vi "Pre Launch Init.vi"(11 "Main Window in":refnum<class "Main Window.lvclass">) -> (0 "error out":errorcluster, 3 "Main Window out":refnum<class "Main Window.lvclass">)   [LabVIEW 2021, in "Recipe.lvlib" / "Main Window.lvclass"]
doc: "Initializes the panel actor. Creates the Panel Helper.\n\n----\nPlease see the following web address for additional documentation and tutorial information:\nhttp://www.mooregoodideas.com/mgi-panel-manager/\n\nAuthor: Derek Trepanier\n\nCopyright (c) 2018, Moore Good Ideas, Inc.\n\nAll rights reserved.\n\nRedistribution and use in source and binary forms, with or without modification, are permitted provided that the following conditions are met:\n\n * Redistributions of source code must retain the above copyright notice, this list of conditions and the following disclaimer.\n * Redistributions in binary form must reproduce the above copyright notice, this list of conditions and the following disclaimer in the documentation and/or other materials provided with the distribution.\n * Neither the name of Moore Good Ideas, Inc. nor the names of its contributors may be used to endorse or promote products derived from this software without specific prior written permission.\n\nTHIS SOFTWARE IS PROVIDED BY THE COPYRIGHT HOLDERS AND CONTRIBUTORS \"AS IS\" AND ANY EXPRESS OR IMPLIED WARRANTIES, INCLUDING, BUT NOT LIMITED TO, THE IMPLIED WARRANTIES OF MERCHANTABILITY AND FITNESS FOR A PARTICULAR PURPOSE ARE DISCLAIMED. IN NO EVENT SHALL THE COPYRIGHT OWNER OR CONTRIBUTORS BE LIABLE FOR ANY DIRECT, INDIRECT, INCIDENTAL, SPECIAL, EXEMPLARY, OR CONSEQUENTIAL DAMAGES (INCLUDING, BUT NOT LIMITED TO, PROCUREMENT OF SUBSTITUTE GOODS OR SERVICES; LOSS OF USE, DATA, OR PROFITS; OR BUSINESS INTERRUPTION) HOWEVER CAUSED AND ON ANY THEORY OF LIABILITY, WHETHER IN CONTRACT, STRICT LIABILITY, OR TORT (INCLUDING NEGLIGENCE OR OTHERWISE) ARISING IN ANY WAY OUT OF THE USE OF THIS SOFTWARE, EVEN IF ADVISED OF THE POSSIBILITY OF SUCH DAMAGE."
uses:
  Main Window.lvclass
  Typedefs/Path--enum.ctl
  <vilib>/MGI/Panel Manager/Panel Actor/Panel Actor/Panel Actor.lvclass
  <vilib>/Thomas ALLIBE/Path Utilities/Path Utilities.lvlib
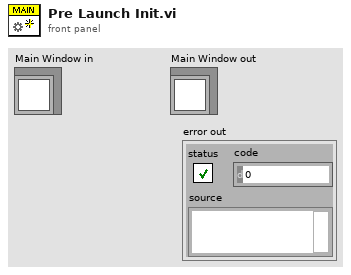
[diagram p1: front panel]
types:
  T1 = typedef "Recipe.lvlib/Main Window.lvclass/Path--enum.ctl" = enum16{"Recipe List File"}
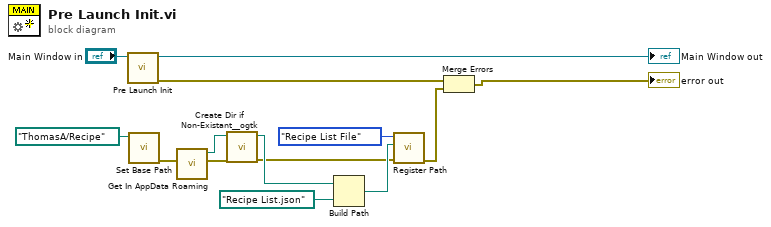
[diagram p0: block diagram]
diagram:
  n1 = call-parent "Pre Launch Init.vi"("Panel Actor in"="Main Window in") -> ("error out"=w14:errorcluster, "Panel Actor out"=→"Main Window out":refnum<class "Main Window.lvclass">)  [unwired: 9 in]
  n2 = call <vilib>:"Set Base Path.vi"("Base Path"=path "ThomasA/Recipe") -> ("error out"=w9:errorcluster)  [unwired: 9 in, 1 out]
  n3 = call <vilib>:"Get In AppData Roaming.vi"("error in (no error)"=w9) -> ("error out"=w5:errorcluster, "Path"=w4:path)  [unwired: 9 in]
  n4 = call <userlib>:"Create Dir if Non-Existant__ogtk.vi"("error in (no error)"=w5, "Directory Path"=w4) -> ("error out"=w2:errorcluster, "dup Directory Path"=w3:path)  [unwired: 7 in, 1 out]
  n5 = Build Path(base path=w3, name or relative path=path "Recipe List.json") -> (appended path=w8:path)
  n6 = call <vilib>:"Register Path.vi"("error in (no error)"=w2, "Path"=w8, "Key"=Path--enum."Recipe List File" ("Path")) -> ("error out"=w10:errorcluster)  [unwired: 6 in, 2 out]
  n7 = Merge Errors(w14, w10) -> (→"error out":errorcluster)
